vi "PathPlanner_TrajectoryState_Interpolate.vi"(9 "Time":dbl, 10 "end Val":T1={"TimeSeconds"=0.0, "VelocityMPS"=0.0, "AccerationMpsSq"=0.0, "HeadingAngularVelRadPerSec"=0.0, "PositionMeters"={"X"=0.0, "Y"=1.0}, "Heading"={"VALUE"=0.0, "COS"=1.0, "SIN"=0.0}, "TargetHolonomicRotation"={"VALUE"=0.0, "COS"=1.0, "SIN"=0.0}, "CurvatureRadPerMeter"=0.0, "PathPlannerConstraints"={"MaxVelocityMps;"=0.0, "MaxAccelerationMpsSq;"=0.0, "MaxAngularVelRadPsEc;"=0.0, "MaxAngularAccRadPSecSq"=0.0, "Exists"=FALSE}, "DeltaPos"=0.0} {"TargetHolonomicRotation"."SIN" format="%13.4f"; "TargetHolonomicRotation"."COS" format="%13.4f"; "TargetHolonomicRotation"."VALUE" format="%13.4f"; "Heading"."SIN" format="%13.4f"; "Heading"."COS" format="%13.4f"; "Heading"."VALUE" format="%13.4f"; "PositionMeters"."Y" format="%14.3f"; "PositionMeters"."X" format="%14.3f"}, 11 "in PathPlannerState":T1={"TimeSeconds"=0.0, "VelocityMPS"=0.0, "AccerationMpsSq"=0.0, "HeadingAngularVelRadPerSec"=0.0, "PositionMeters"={"X"=0.0, "Y"=1.0}, "Heading"={"VALUE"=0.0, "COS"=1.0, "SIN"=0.0}, "TargetHolonomicRotation"={"VALUE"=0.0, "COS"=1.0, "SIN"=0.0}, "CurvatureRadPerMeter"=0.0, "PathPlannerConstraints"={"MaxVelocityMps;"=0.0, "MaxAccelerationMpsSq;"=0.0, "MaxAngularVelRadPsEc;"=0.0, "MaxAngularAccRadPSecSq"=0.0, "Exists"=FALSE}, "DeltaPos"=0.0} {"TargetHolonomicRotation"."SIN" format="%13.4f"; "TargetHolonomicRotation"."COS" format="%13.4f"; "TargetHolonomicRotation"."VALUE" format="%13.4f"; "Heading"."SIN" format="%13.4f"; "Heading"."COS" format="%13.4f"; "Heading"."VALUE" format="%13.4f"; "PositionMeters"."Y" format="%14.3f"; "PositionMeters"."X" format="%14.3f"}) -> (3 "interpolated PathPlanner State":T1={"TimeSeconds"=0.0, "VelocityMPS"=0.0, "AccerationMpsSq"=0.0, "HeadingAngularVelRadPerSec"=0.0, "PositionMeters"={"X"=0.0, "Y"=1.0}, "Heading"={"VALUE"=0.0, "COS"=1.0, "SIN"=0.0}, "TargetHolonomicRotation"={"VALUE"=0.0, "COS"=1.0, "SIN"=0.0}, "CurvatureRadPerMeter"=0.0, "PathPlannerConstraints"={"MaxVelocityMps;"=0.0, "MaxAccelerationMpsSq;"=0.0, "MaxAngularVelRadPsEc;"=0.0, "MaxAngularAccRadPSecSq"=0.0, "Exists"=FALSE}, "DeltaPos"=0.0} {"TargetHolonomicRotation"."SIN" format="%13.4f"; "TargetHolonomicRotation"."COS" format="%13.4f"; "TargetHolonomicRotation"."VALUE" format="%13.4f"; "Heading"."SIN" format="%13.4f"; "Heading"."COS" format="%13.4f"; "Heading"."VALUE" format="%13.4f"; "PositionMeters"."Y" format="%14.3f"; "PositionMeters"."X" format="%14.3f"})   [LabVIEW 2019, in "PathPlanner.lvlib"]
doc: "Interpolate between this state and the given state\n \nInputs: \n - trajectoryState - cluster - this trajectory state\n - endVal - cluster - State to interpolate with\n - t - double - Interpolation factor (0.0-1.0)\n\nOutputs:\n - Interpolated state - trajectory state - interpolated state"
uses:
  PathPlanner.lvlib
  TypeDef/PathPlannerTrajectoryState.ctl
  <vilib>/Rock Robotics/WPI/ThirdParty/JAS_Junk/TrajLib/TypeDef/TRANSLATION2D.ctl
  <vilib>/Rock Robotics/WPI/ThirdParty/JAS_Junk/TrajLib/TypeDef/ROTATION2D.ctl
  TypeDef/PathPlannerPathConstraints.ctl
  <vilib>/Rock Robotics/WPI/ThirdParty/JAS_Junk/TrajLib/Translation2d_Create.vi
  <vilib>/Rock Robotics/WPI/ThirdParty/JAS_Junk/TrajLib/MathUtil_Interpolate.vi
  <vilib>/Rock Robotics/WPI/ThirdParty/JAS_Junk/TrajLib/Translation2d_GetXY.vi
  <vilib>/Rock Robotics/WPI/ThirdParty/JAS_Junk/TrajLib/Rotation2d_Plus.vi
  <vilib>/Rock Robotics/WPI/ThirdParty/JAS_Junk/TrajLib/Rotation2d_Minus.vi
  <vilib>/Rock Robotics/WPI/ThirdParty/JAS_Junk/TrajLib/MathUtil_Clamp.vi
  <vilib>/Rock Robotics/WPI/ThirdParty/JAS_Junk/TrajLib/Rotation2d_Times.vi
  <vilib>/Rock Robotics/WPI/ThirdParty/JAS_Junk/TrajLib/Rotation2d_RotateBy.vi
  <vilib>/Rock Robotics/WPI/ThirdParty/JAS_Junk/TrajLib/Rotation2d_UnaryMinus.vi
  <vilib>/Rock Robotics/WPI/ThirdParty/JAS_Junk/TrajLib/Rotation2d_CreateAngle.vi
  <vilib>/Rock Robotics/WPI/ThirdParty/JAS_Junk/TrajLib/Rotation2d_CreateXY.vi
  <vilib>/Rock Robotics/WPI/ThirdParty/JAS_Junk/TrajLib/Util_CalcDist.vi
  <vilib>/Rock Robotics/WPI/ThirdParty/JAS_Junk/TrajLib/Trajectory_Library.lvlib
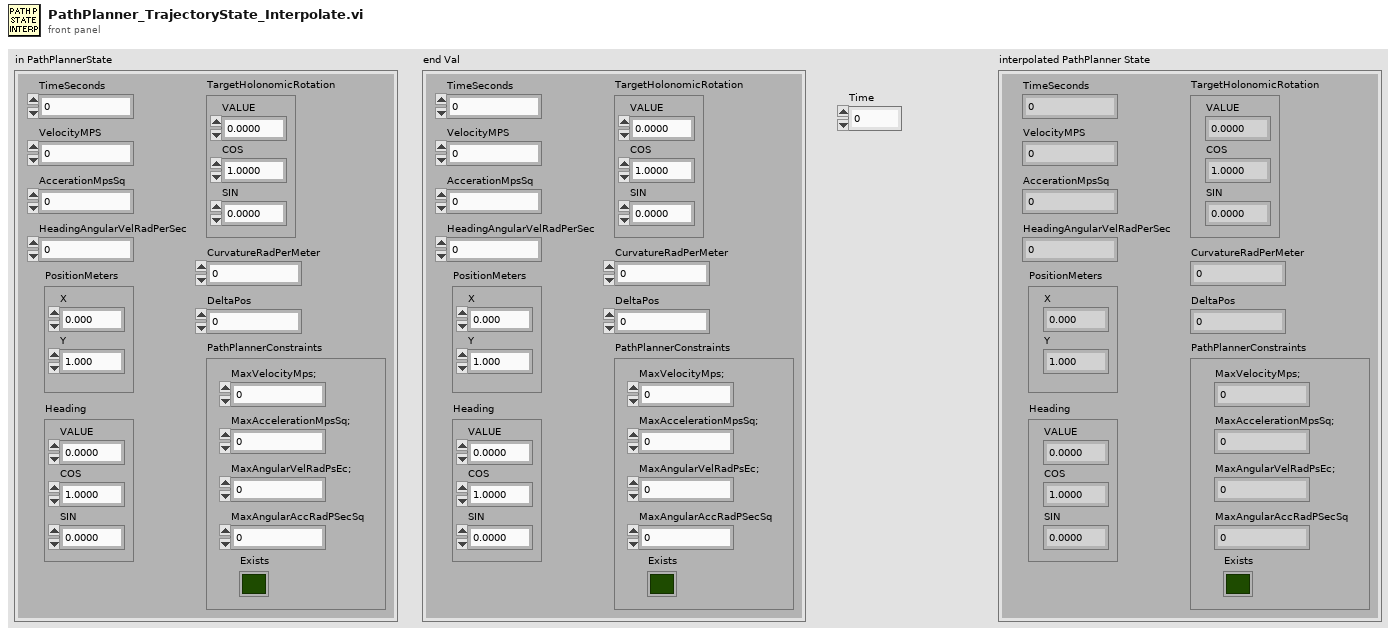
[diagram p1: front panel]
types:
  T1 = typedef "PathPlanner.lvlib/PathPlannerTrajectoryState.ctl" = cluster{"TimeSeconds":dbl, "VelocityMPS":dbl, "AccerationMpsSq":dbl, "HeadingAngularVelRadPerSec":dbl, "PositionMeters":T2, "Heading":T3, "TargetHolonomicRotation":T3, "CurvatureRadPerMeter":dbl, "PathPlannerConstraints":T4, "DeltaPos":dbl}
  T2 = typedef "Trajectory_Library.lvlib/TRANSLATION2D.ctl" = cluster{"X":dbl, "Y":dbl}
  T3 = typedef "Trajectory_Library.lvlib/ROTATION2D.ctl" = cluster{"VALUE":dbl, "COS":dbl, "SIN":dbl}
  T4 = typedef "PathPlanner.lvlib/PathPlannerPathConstraints.ctl" = cluster{"MaxVelocityMps;":dbl, "MaxAccelerationMpsSq;":dbl, "MaxAngularVelRadPsEc;":dbl, "MaxAngularAccRadPSecSq":dbl, "Exists":bool}
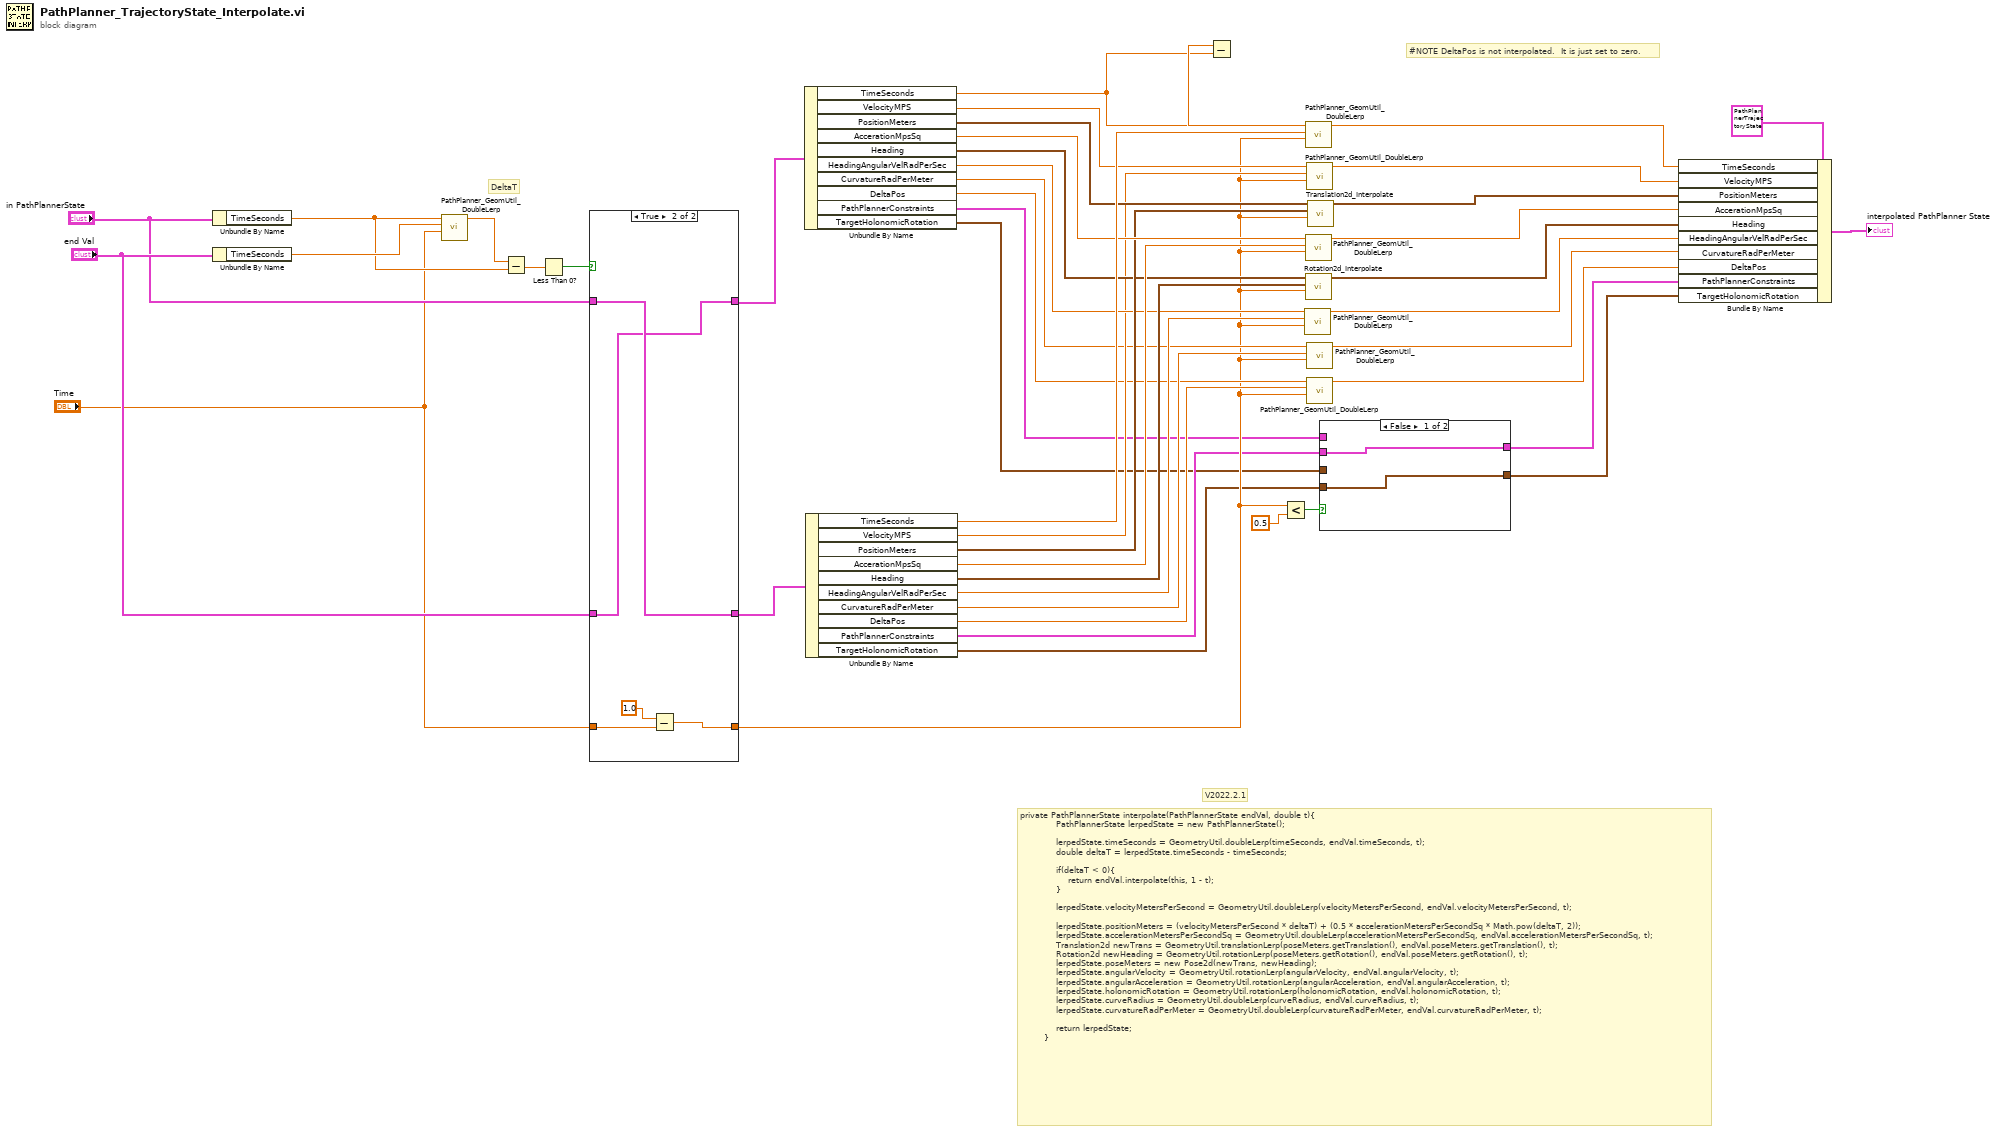
[diagram p0: block diagram]
diagram:
  # "DeltaT"
  # "V2022.2.1"
  # "private PathPlannerState interpolate(PathPlannerState endVal, double t){\n            PathPlannerState lerpedState = new PathPlannerState();\n\n            lerpedState.timeSeconds = GeometryUtil.doubleLerp(timeSeconds, endVal.timeSeconds, t);\n            double deltaT = lerpedState.timeSeconds - timeSeconds;\n\n            if(deltaT < 0){\n                return endVal.interpolate(this, 1 - t);\n            }\n\n            lerpedState.velocityMetersPerSecond = GeometryUtil.doubleLerp(velocityMetersPerSecond, endVal.velocityMetersPerSecond, t);\n\n            lerpedState.positionMeters = (velocityMetersPerSecond * deltaT) + (0.5 * accelerationMetersPerSecondSq * Math.pow(deltaT, 2));\n            lerpedState.accelerationMetersPerSecondSq = GeometryUtil.doubleLerp(accelerationMetersPerSecondSq, endVal.accelerationMetersPerSecondSq, t);\n            Translation2d newTrans = GeometryUtil.translationLerp(poseMeters.getTranslation(), endVal.poseMeters.getTranslation(), t);\n            Rotation2d newHeading = GeometryUtil.rotationLerp(poseMeters.getRotation(), endVal.poseMeters.getRotation(), t);\n            lerpedState.poseMeters = new Pose2d(newTrans, newHeading);\n            lerpedState.angularVelocity = GeometryUtil.rotationLerp(angularVelocity, endVal.angularVelocity, t);\n            lerpedState.angularAcceleration = GeometryUtil.rotationLerp(angularAcceleration, endVal.angularAcceleration, t);\n            lerpedState.holonomicRotation = GeometryUtil.rotationLerp(holonomicRotation, endVal.holonomicRotation, t);\n            lerpedState.curveRadius = GeometryUtil.doubleLerp(curveRadius, endVal.curveRadius, t);\n            lerpedState.curvatureRadPerMeter = GeometryUtil.doubleLerp(curvatureRadPerMeter, endVal.curvatureRadPerMeter, t);\n\n            return lerpedState;\n        }"
  # "#NOTE DeltaPos is not interpolated.  It is just set to zero."
  n1 = Unbundle By Name("in PathPlannerState") -> ("TimeSeconds"=w41:dbl)
  n2 = Unbundle By Name("end Val") -> ("TimeSeconds"=w43:dbl)
  n3 = call "PathPlanner_GeomUtil_DoubleLerp.vi"("T"="Time", "EndVal"=w43, "StartVal"=w41) -> ("Lerp"=w42:dbl)  [unwired: 8 in]
  n4 = Subtract(x=w42, y=w41) -> (x-y=w40:dbl)
  n5 = Less Than 0?(x=w40) -> (x < 0?=w39:bool)
  n6 = case shown="True" w39 {
    tunnel: "end Val" -> [w48 w52]
    tunnel: [w48 w53] -> w34
    tunnel: "in PathPlannerState" -> [w47 w53]
    tunnel: [w47 w52] -> w35
    tunnel: [w46 w49] -> w9
    tunnel: "Time" -> [w46 w50]
    frame False {
    }
    frame True {
      n7 = Subtract(x=1.0, y=w50) -> (x-y=w49:dbl)
    }
  }
  n8 = Unbundle By Name(w35) -> ("TimeSeconds"=w31:dbl, "VelocityMPS"=w27:dbl, "PositionMeters"=w26:T2, "AccerationMpsSq"=w30:dbl, "Heading"=w22:T3, "HeadingAngularVelRadPerSec"=w19:dbl, "CurvatureRadPerMeter"=w15:dbl, "DeltaPos"=w12:dbl, "PathPlannerConstraints"=w6:T4, "TargetHolonomicRotation"=w3:T3)
  n9 = Unbundle By Name(w34) -> ("TimeSeconds"=w33:dbl, "VelocityMPS"=w18:dbl, "PositionMeters"=w24:T2, "AccerationMpsSq"=w25:dbl, "Heading"=w21:T3, "HeadingAngularVelRadPerSec"=w17:dbl, "CurvatureRadPerMeter"=w14:dbl, "DeltaPos"=w11:dbl, "PathPlannerConstraints"=w5:T4, "TargetHolonomicRotation"=w2:T3)
  n10 = Less?(x=w9, y=0.5) -> (x < y?=w7:bool)
  n11 = call "PathPlanner_GeomUtil_DoubleLerp.vi"("T"=w9, "EndVal"=w17, "StartVal"=w19) -> ("Lerp"=w16:dbl)  [unwired: 8 in]
  n12 = call "PathPlanner_GeomUtil_DoubleLerp.vi"("T"=w9, "EndVal"=w33, "StartVal"=w31) -> ("Lerp"=w32:dbl)  [unwired: 8 in]
  n13 = Subtract(x=w32, y=w31) -> ()  [unwired: 1 out]
  n14 = call "PathPlanner_GeomUtil_DoubleLerp.vi"("T"=w9, "EndVal"=w25, "StartVal"=w30) -> ("Lerp"=w29:dbl)  [unwired: 8 in]
  n15 = call <vilib>:"Rotation2d_Interpolate.vi"("T"=w9, "EncValue ROTATION"=w21, "in ROTATION"=w22) -> ("Interpolated ROTATION"=w20:T3)  [unwired: 8 in]
  n16 = call "PathPlanner_GeomUtil_DoubleLerp.vi"("T"=w9, "EndVal"=w18, "StartVal"=w27) -> ("Lerp"=w28:dbl)  [unwired: 8 in]
  n17 = call "PathPlanner_GeomUtil_DoubleLerp.vi"("T"=w9, "EndVal"=w14, "StartVal"=w15) -> ("Lerp"=w13:dbl)  [unwired: 8 in]
  n18 = call "PathPlanner_GeomUtil_DoubleLerp.vi"("T"=w9, "EndVal"=w11, "StartVal"=w12) -> ("Lerp"=w10:dbl)  [unwired: 8 in]
  n19 = call <vilib>:"Translation2d_Interpolate.vi"("T"=w9, "other Translation"=w24, "In Translation"=w26) -> ("Interpolated Translation"=w23:T2)  [unwired: 8 in]
  n20 = case shown="False" w7 {
    tunnel: w6 -> [_ w57]
    tunnel: w5 -> [w55 _]
    tunnel: [w55 w57] -> w4
    tunnel: w3 -> [_ w56]
    tunnel: w2 -> [w54 _]
    tunnel: [w54 w56] -> w1
    frame False {
    }
    frame True {
    }
  }
  n21 = Bundle By Name(cluster=T1 {"TimeSeconds"=0.0, "VelocityMPS"=0.0, "AccerationMpsSq"=0.0, "HeadingAngularVelRadPerSec"=0.0, "PositionMeters"={"X"=0.0, "Y"=1.0}, "Heading"={"VALUE"=0.0, "COS"=1.0, "SIN"=0.0}, "TargetHolonomicRotation"={"VALUE"=0.0, "COS"=1.0, "SIN"=0.0}, "CurvatureRadPerMeter"=0.0, "PathPlannerConstraints"={"MaxVelocityMps;"=0.0, "MaxAccelerationMpsSq;"=0.0, "MaxAngularVelRadPsEc;"=0.0, "MaxAngularAccRadPSecSq"=0.0, "Exists"=FALSE}, "DeltaPos"=0.0} ("PathPlannerState"), "TimeSeconds"=w32, "VelocityMPS"=w28, "PositionMeters"=w23, "AccerationMpsSq"=w29, "Heading"=w20, "HeadingAngularVelRadPerSec"=w16, "CurvatureRadPerMeter"=w13, "DeltaPos"=w10, "PathPlannerConstraints"=w4, "TargetHolonomicRotation"=w1) -> (→"interpolated PathPlanner State":T1)
